vi "WriteData.vi"(8 "error in (no error)":errorcluster, 10 "DataToWrite":string, 11 "Communication in":refnum<class "Communication.lvclass">) -> (0 "error out":errorcluster, 3 "Communication out":refnum<class "Communication.lvclass">)   [LabVIEW 2019, in "Communication.lvclass"]
uses:
  Communication.lvclass
  Communication.lvclass/Communication.ctl
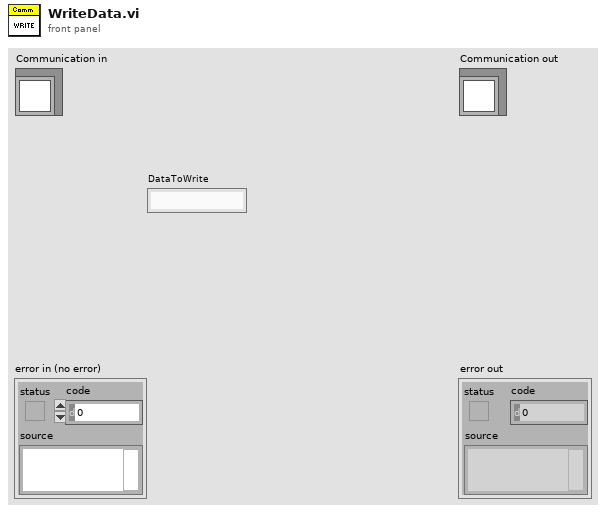
[diagram p1: front panel]
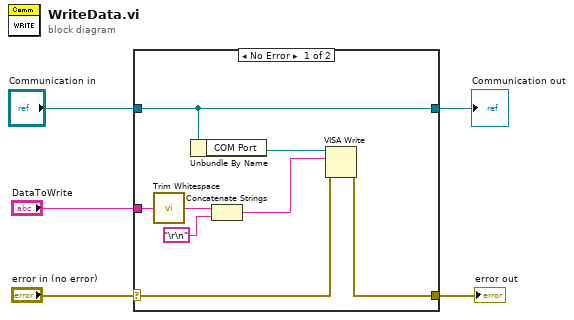
[diagram p0: block diagram]
diagram:
  n1 = case shown="No Error" "error in (no error)" {
    selector: "error in (no error)" -> [w12 w15]
    tunnel: [w8 w15] -> w4
    tunnel: [w9 w14] -> w2
    tunnel: "Communication in" -> [w9 w14]
    tunnel: "DataToWrite" -> [w11 _]
    frame No Error {
      n2 = call <vilib>:"Trim Whitespace.vi"("string"=w11) -> ("trimmed string"=w6:string)  [unwired: 1 in]
      n3 = Unbundle By Name(w9) -> ("COM Port"=w13:refnum<visa-resource-name>)
      n4 = Concatenate Strings(w6, "\r\n") -> (w7:string)
      n5 = VISA Write(VISA resource name=w13, write buffer=w7, error in (no error)=w12) -> (error out=w8:errorcluster)  [unwired: 2 out]
    }
    frame Error {
    }
  }
  "error out" <- w4
  "Communication out" <- w2
